vi "Create Transport DAT File.vi"(6 "append to existing file?\n(new file:F)":bool, 8 "error in (no error)":errorcluster, 10 "Wavenames":string[](array[string]), 11 "Control Experiment in":refnum<class "Control Experiment.lvclass">) -> (0 "error out":errorcluster, 3 "Control Experiment out":refnum<class "Control Experiment.lvclass">)   [LabVIEW 2016, in "Control Experiment.lvclass"]
uses:
  Control Experiment.lvclass
  Control Experiment.lvclass/Control Experiment.ctl
  <userlib>/LevyLab/LV to ITX/LVtoITX.lvclass
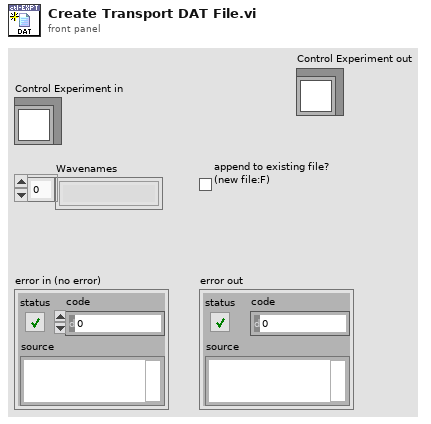
[diagram p1: front panel]
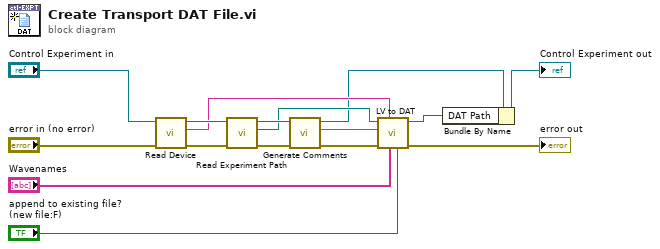
[diagram p0: block diagram]
diagram:
  n1 = call "Read Device.vi"("error in (no error)"="error in (no error)", "Control Experiment in"="Control Experiment in") -> ("error out"=w11:errorcluster, "Device"=w5:string, "Control Experiment out"=w7:refnum<class "Control Experiment.lvclass">)  [unwired: 7 in]
  n2 = call "Read Experiment Path.vi"("error in (no error)"=w11, "Control Experiment in"=w7) -> ("error out"=w10:errorcluster, "Experiment Path"=w4:path, "Control Experiment out"=w8:refnum<class "Control Experiment.lvclass">)  [unwired: 7 in]
  n3 = call "Generate Comments.vi"("error in (no error)"=w10, "Control Experiment"=w8) -> ("error out"=w9:errorcluster, "Comments"=w6:string, "Control Experiment out"=w2:refnum<class "Control Experiment.lvclass">)  [unwired: 6 in]
  n4 = call <userlib>:"LV to DAT.vi"("append to file? (new file:F)"="append to existing file?\n(new file:F)", "wavenames (.Vx, etc)"="Wavenames", "filename"=w5, "error in"=w9, "Comments"=w6, "path"=w4) -> ("error out"=→"error out":errorcluster, "new file path"=w3:path)  [unwired: 4 in]
  n5 = Bundle By Name(cluster=w2, "DAT Path"=w3) -> (→"Control Experiment out":refnum<class "Control Experiment.lvclass">)
